vi "protectionSD.vi"(4 "current Alarm break, uA":dbl=100.0 format="%#_13g", 5 "Block accelerator":refnum<vi>, 6 "current Alarm, uA":dbl=1000.0 format="%#_13g", 7 "Accelerator protected":refnum<vi>, 8 "error in (no error)":errorcluster, 9 "cluster of DAQ tasks":T1, 10 "Alarm Refnum":refnum<vi>, 11 "Relay key refnum":refnum<vi>) -> (0 "error out":errorcluster, 1 "Alarm current":dbl)   [LabVIEW 2015]
uses:
  controls/Daqmxtasks.ctl
  <vilib>/DAQmx/read.llb/DAQmx Read (Analog 1D DBL 1Chan NSamp).vi
  <vilib>/Analysis/baseanly.llb/Mean (DBL).vi
  <vilib>/DAQmx/write.llb/DAQmx Write (Digital Bool 1Line 1Point).vi
  <vilib>/DAQmx/read.llb/DAQmx Read (Digital Bool 1Line 1Point).vi
  <vilib>/DAQmx/miscellaneous.llb/DAQmx Fill In Error Info.vi
  globalVarSD.vi
  <vilib>/Analysis/NI_AALBase.lvlib
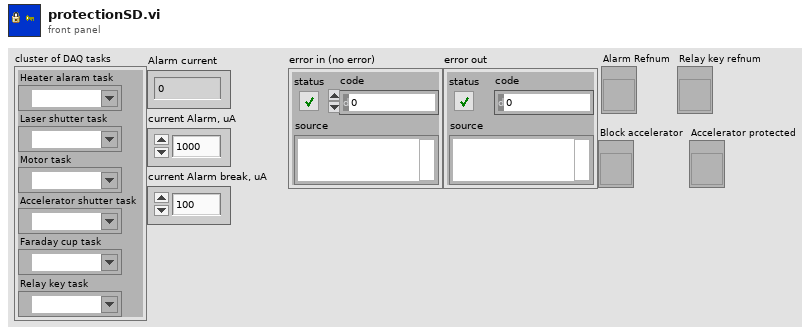
[diagram p1: front panel]
types:
  T1 = typedef "Daqmxtasks.ctl" = cluster{"Heater alaram task":refnum<k21>, "Laser shutter task":refnum<k21>, "Motor task":refnum<k21>, "Accelerator shutter task":refnum<k21>, "Relay key task":refnum<k21>, "Faraday cup task":refnum<k21>}
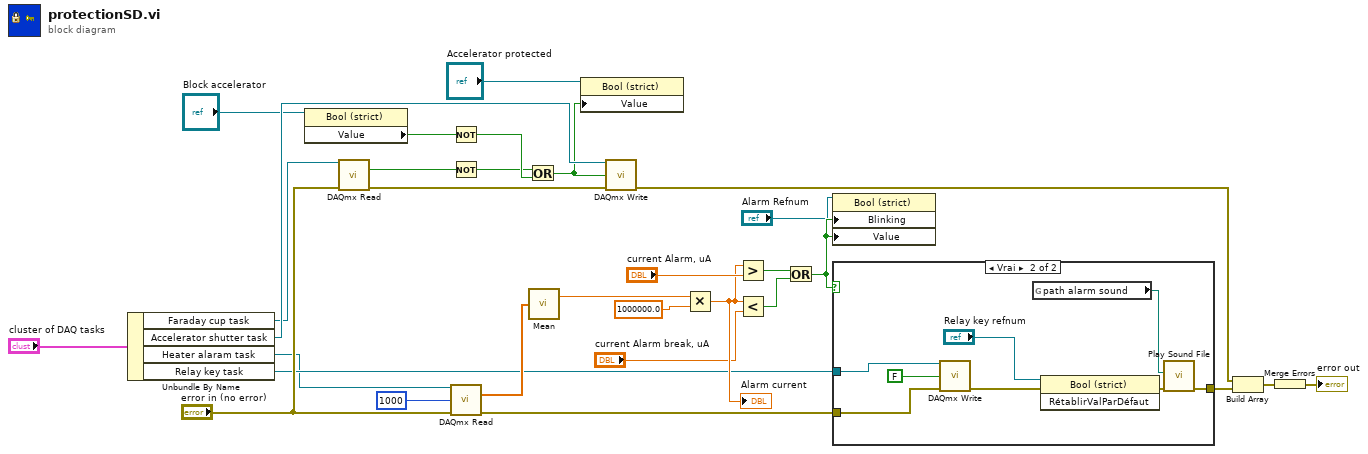
[diagram p0: block diagram]
diagram:
  n1 = Unbundle By Name("cluster of DAQ tasks") -> ("Faraday cup task"=w7:refnum<k21>, "Accelerator shutter task"=w8:refnum<k21>, "Heater alaram task"=w9:refnum<k21>, "Relay key task"=w10:refnum<k21>)
  n2 = property on="Property Node" class="Bool (strict)"(reference="Block accelerator") -> ("Value"=w1:bool)  [unwired: 1 in, 2 out]
  n3 = call-poly <vilib>:"DAQmx Read.vi"("task/channels in"=w7, "error in"="error in (no error)") -> ("data"=w26:bool, "error out"=w27:errorcluster)  [unwired: 11 in, 1 out]
  n4 = Not(x=w1) -> (.not. x?=w25:bool)
  n5 = Not(x=w26) -> (.not. x?=w24:bool)
  n6 = call-poly <vilib>:"DAQmx Read.vi"("task/channels in"=w9, "number of samples per channel"=1000, "error in"="error in (no error)") -> ("data"=w22:dbl[], "error out"=w17:errorcluster)  [unwired: 10 in, 1 out]
  n7 = Or(x=w24, y=w25) -> (x .or. y?=w3:bool)
  n8 = call-poly <vilib>:"Mean.vi"("X"=w22) -> ("mean"=w21:dbl)  [unwired: 1 out]
  n9 = property on="Property Node" class="Bool (strict)"(reference="Accelerator protected", "Value"=w3) -> ()  [unwired: 1 in, 2 out]
  n10 = call-poly <vilib>:"DAQmx Write.vi"("task/channels in"=w8, "data"=w3, "error in"=w27) -> ("error out"=w19:errorcluster)  [unwired: 10 in, 2 out]
  n11 = Multiply(x=w21, y=1000000.0) -> (x*y=w14:dbl)
  "Alarm current" <- w14
  n12 = Greater?(x=w14, y="current Alarm, uA") -> (0:w12:bool)
  n13 = Less?(x=w14, y="current Alarm break, uA") -> (x < y?=w11:bool)
  n14 = Or(x=w12, y=w11) -> (x .or. y?=w6:bool)
  n15 = property on="Property Node" class="Bool (strict)"(reference="Alarm Refnum", "Blinking"=w6, "Value"=w6) -> ()  [unwired: 1 in, 2 out]
  n16 = case shown="Vrai" w6 {
    tunnel: w17 -> [w31 w38]
    tunnel: [w31 w39] -> w16
    tunnel: w10 -> [_ w37]
    frame False {
    }
    frame True {
      n17 = call-poly <vilib>:"DAQmx Write.vi"("task/channels in"=w37, "data"=FALSE, "error in"=w38) -> ("error out"=w35:errorcluster)  [unwired: 10 in, 2 out]
      n18 = global read "globalVarSD.vi" "path alarm sound"() -> (w33:path)
      n19 = invoke on="Invoke Node" class="Bool (strict)" method="RétablirValParDéfaut"(reference="Relay key refnum", error in=w35) -> (error out=w34:errorcluster)  [unwired: 1 in, 2 out]
      n20 = call <vilib>:"Play Sound File.vi"("error in (no error)"=w34, "path"=w33) -> ("error out"=w39:errorcluster)  [unwired: 8 in, 1 out]
    }
  }
  n21 = Build Array(w19, w16) -> (w18:errorcluster[])
  n22 = Merge Errors(w18) -> (→"error out":errorcluster)
